vi "is_done.vi"(8 "error in (no error)":errorcluster, 11 "DAQmx_pulse_out in":refnum<class "DAQmx_pulse_out.lvclass">) -> (0 "error out":errorcluster, 2 "task done?":bool, 3 "DAQmx_pulse_out out":refnum<class "DAQmx_pulse_out.lvclass">)   [LabVIEW 2013, in "DAQmx_pulse_out.lvclass"]
uses:
  DAQmx_pulse_out.lvclass
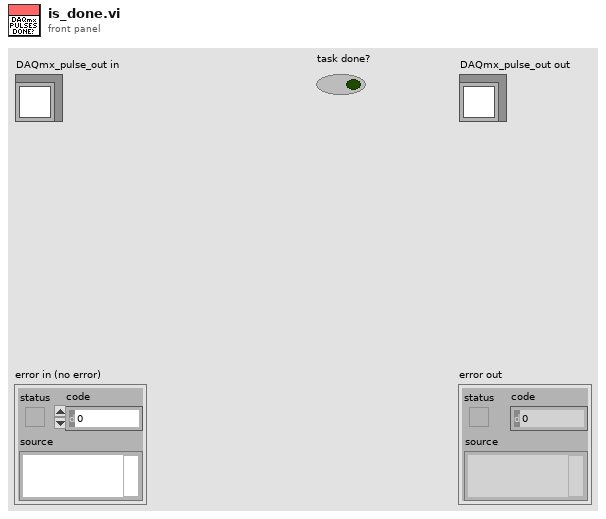
[diagram p1: front panel]
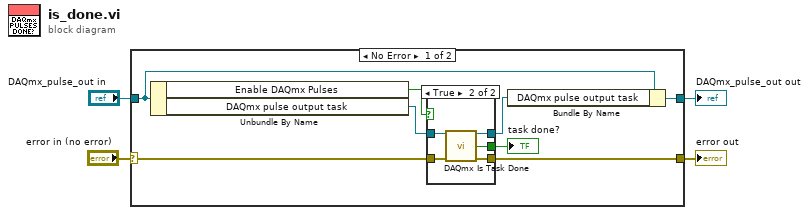
[diagram p0: block diagram]
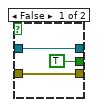
[diagram p2: hidden frame]
diagram:
  n1 = case shown="No Error" "error in (no error)" {
    selector: "error in (no error)" -> [w11 w22]
    tunnel: [w10 w22] -> w3
    tunnel: [w7 w21] -> w1
    tunnel: "DAQmx_pulse_out in" -> [w8 w21]
    frame No Error {
      n2 = Unbundle By Name(w8) -> ("Enable DAQmx Pulses"=w12:bool, "DAQmx pulse output task"=w9:refnum<k21>)
      n3 = case shown="True" w12 {
        tunnel: w11 -> [w15 w20]
        tunnel: [w15 w19] -> w10
        tunnel: w9 -> [w14 w18]
        tunnel: [w14 w17] -> w6
        tunnel: [TRUE ("task done?") w16] -> w5
        frame False {
        }
        frame True {
          n4 = call <vilib>:"DAQmx Is Task Done.vi"("task/channels in"=w18, "error in"=w20) -> ("task out"=w17:refnum<k21>, "task done?"=w16:bool, "error out"=w19:errorcluster)  [unwired: 11 in]
        }
      }
      "task done?" <- w5
      n5 = Bundle By Name(cluster=w8, "DAQmx pulse output task"=w6) -> (w7:refnum<class "DAQmx_pulse_out.lvclass">)
    }
    frame Error {
    }
  }
  "error out" <- w3
  "DAQmx_pulse_out out" <- w1
